vi "Channel Count.vi"(8 "error in (no error)":errorcluster, 11 "Transfer Configuration in":refnum<class "Transfer Configuration.lvclass">) -> (0 "error out":errorcluster, 2 "total channel count":u64, 3 "Transfer Configuration out":refnum<class "Transfer Configuration.lvclass">)   [LabVIEW 2017, in "Data Sharing Framework Engine.lvlib" / "Transfer Configuration.lvclass"]
uses:
  Transfer Configuration.lvclass
  Transfer Configuration.lvclass/Transfer Configuration.ctl
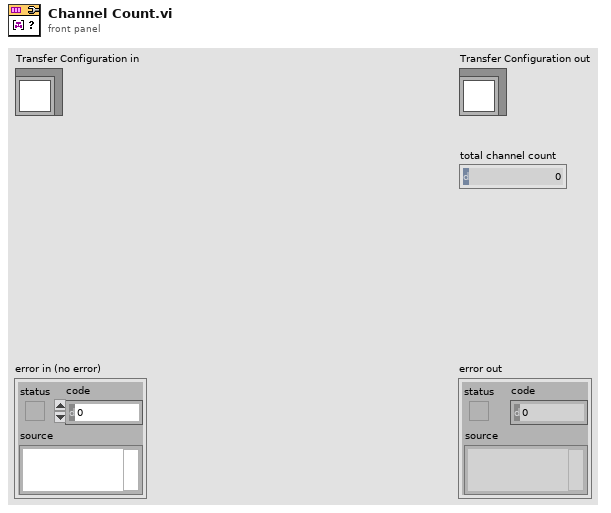
[diagram p1: front panel]
types:
  T1 = typedef "Data Sharing Framework Engine.lvlib/DSF Runtime Channel Block.ctl" = cluster{"data type":T2, "count":u64, "buffer offset":u64}
  T2 = typedef "DSF Configuration API.lvlib/DSF Data Type.ctl" = enum8{"Bool", "SGL", "DBL", "I8", "I16", "I32", "I64", "U8", "U16", "U32", "U64"}
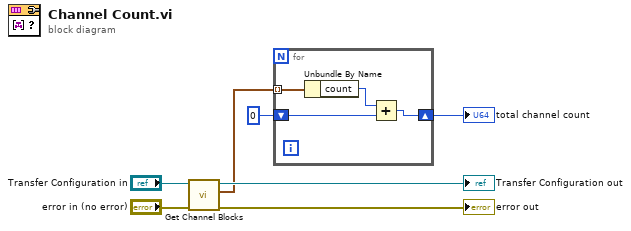
[diagram p0: block diagram]
diagram:
  n1 = call "Get Channel Blocks.vi"("Transfer Configuration in"="Transfer Configuration in") -> ("channel blocks"=w3:T1[], "Transfer Configuration out"=→"Transfer Configuration out":refnum<class "Transfer Configuration.lvclass">)  [unwired: 9 in]
  n2 = for {
    tunnel: w3 -> [w10] mode=indexing
    shift-right: [w7] -> w1
    shift-left: u64 0 -> [w9]
    n3 = Unbundle By Name(w10) -> ("count"=w8:u64)
    n4 = Add(x=w8, y=w9) -> (x+y=w7:u64)
  }
  "total channel count" <- w1
  "error out" <- "error in (no error)"
